vi "FTW-Endpoint-Bind.vi"(0 "FTW Endpoint":refnum<class "FTW-Endpoint.lvclass">, 5 "Endpoint Address":T1, 7 "Requested Identity":string, 11 "error in":errorcluster) -> (4 "FTW Endpoint out":refnum<class "FTW-Endpoint.lvclass">, 6 "Actual Endpoint Address":T1, 8 "Actual Identity":string, 15 "error out":errorcluster)   [LabVIEW 2012, in "FTW-Actor.lvlib" / "FTW-Endpoint.lvclass"]
uses:
  FTW-Endpoint.lvclass
  Utility/FTW-Actor-Address.ctl
  FTW-Endpoint.lvclass/FTW-Endpoint.ctl
  FTW-Actor.lvlib
panel:
  # "Inputs"
  # "Outputs"
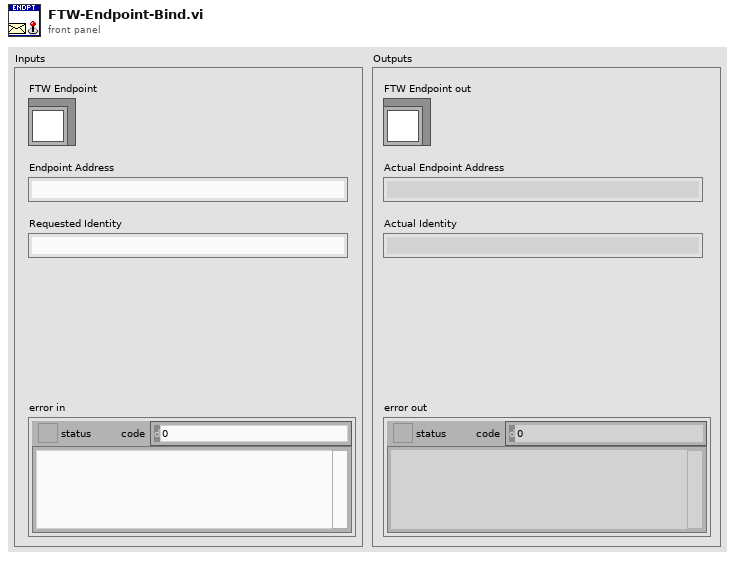
[diagram p1: front panel]
types:
  T1 = typedef "FTW-Actor.lvlib/FTW-Actor-Address.ctl" = string
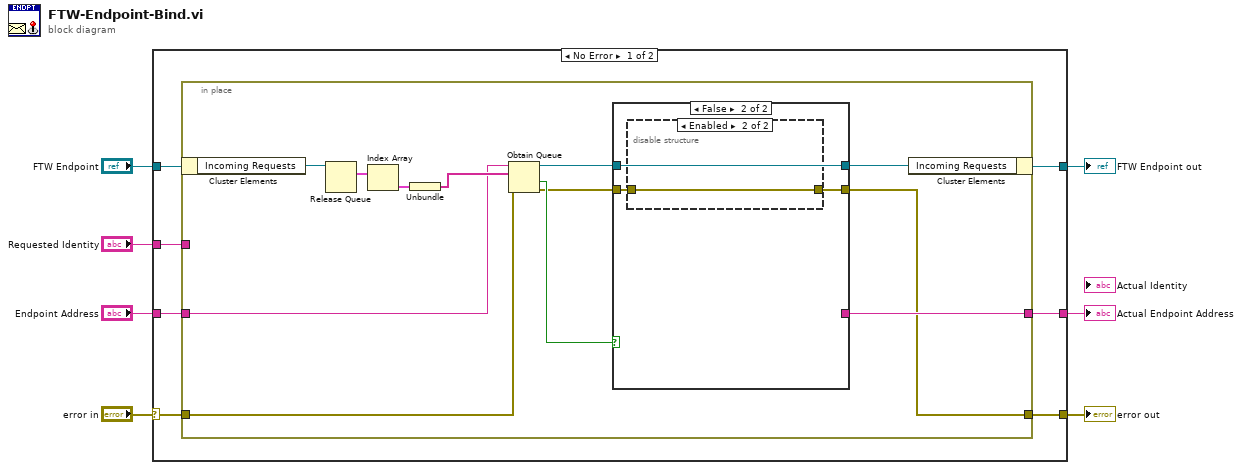
[diagram p0: block diagram]
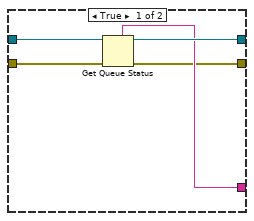
[diagram p2: hidden frame]
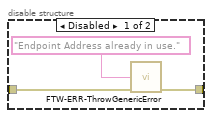
[diagram p3: hidden frame]
diagram:
  n1 = case shown="No Error" "error in" {
    selector: "error in" -> [w12 w40]
    tunnel: [w8 w40] -> w7
    tunnel: [w9 w39] -> w5
    tunnel: "FTW Endpoint" -> [w14 w39]
    tunnel: "Requested Identity" -> [w13 _]
    tunnel: "Endpoint Address" -> [w11 _]
    tunnel: [w10 _] -> w1
    frame No Error {
      n2 = in-place {
        in-place-border: w13 -> [_]
        in-place-border: w12 -> [w22]
        in-place-border: [w15] -> w8
        in-place-border: w11 -> [w19]
        in-place-border: [w20] -> w10
        n3 = in-place-cluster #1(w14) -> ("Incoming Requests"=w26:refnum<queue>)
        n4 = Release Queue(queue=w26) -> (remaining elements=w25:cluster{"Multipart Message":string[]}[])  [unwired: 2 in, 2 out]
        n5 = Index Array(array=w25) -> (element=w24:cluster{"Multipart Message":string[]})  [unwired: 1 in]
        n6 = Unbundle(w24) -> ("Multipart Message"=w23:string[])
        n7 = Obtain Queue(name (unnamed)=w19, element data type=w23, error in (no error)=w22) -> (queue out=w17:refnum<queue>, created new?=w21:bool, error out=w16:errorcluster)  [unwired: 2 in]
        n8 = case shown="False" w21 {
          tunnel: [w28 _] -> w20
          tunnel: [w30 w33] -> w18
          tunnel: w17 -> [w31 w33]
          tunnel: w16 -> [w29 w34]
          tunnel: [w27 w32] -> w15
          frame True {
            n9 = Get Queue Status(queue=w31, error in (no error)=w29) -> (queue out=w30:refnum<queue>, queue name=w28:string, error out=w27:errorcluster)  [unwired: 1 in, 5 out]
          }
          frame False {
            n10 = disable-structure shown="Enabled" {
              disable-tunnel: w34 -> [w37 w38]
              disable-tunnel: [w36 w38] -> w32
              frame Disabled {
                n11 = call "FTW-ERR-ThrowGenericError.vi"("Error Message"="Endpoint Address already in use.", "error in"=w37) -> ("error out"=w36:errorcluster)  [unwired: 13 in]
              }
              frame Enabled {
              }
            }
          }
        }
        n12 = in-place-cluster #1("Incoming Requests"=w18) -> (w9:refnum<class "FTW-Endpoint.lvclass">)
      }
    }
    frame Error {
    }
  }
  "error out" <- w7
  "FTW Endpoint out" <- w5
  "Actual Endpoint Address" <- w1
